vi "Cycle Complete.vi"(8 "error in (no error)":errorcluster, 11 "Active in":refnum<class "Active.lvclass">) -> (0 "error out":errorcluster, 3 "_State Machine Actor out":refnum<class "_State Machine Actor.lvclass">)   [LabVIEW 2024, in "Active.lvlib" / "Active.lvclass"]
uses:
  Active.lvclass
  Active.lvclass/Active.ctl
  Idle/Idle/Idle.lvclass
  C:/Users/uspoaotto/OneDrive - Oregon Tool/Desktop/working copies/stateMachineActor/src/Automation Controller/Automation Controller/Automation Controller.lvclass
  C:/Users/uspoaotto/OneDrive - Oregon Tool/Desktop/working copies/stateMachineActor/src/State Machine Actor/State Machine Actor/State Machine Actor.lvclass
  C:/Users/uspoaotto/OneDrive - Oregon Tool/Desktop/working copies/stateMachineActor/src/_State Machine Actor/_State Machine Actor/_State Machine Actor.lvclass
  C:/Program Files (x86)/National Instruments/LabVIEW 2024/vi.lib/ActorFramework/Actor/Actor.lvclass
  C:/Users/uspoaotto/OneDrive - Oregon Tool/Desktop/working copies/stateMachineActor/src/Idle/Idle/Idle.lvclass
  _State Machine Actor/_State Machine Actor/_State Machine Actor.lvclass
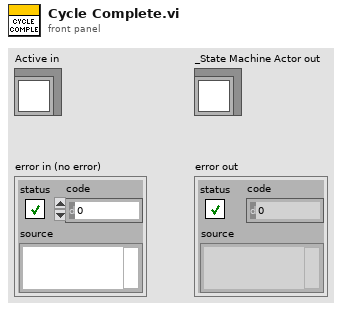
[diagram p1: front panel]
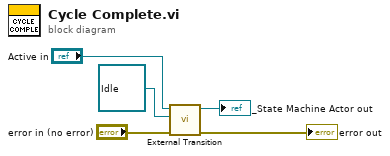
[diagram p0: block diagram]
diagram:
  n1 = call-dynamic "External Transition.vi"("error in (no error)"="error in (no error)", "Target State"=refnum<class "Idle.lvclass"> refnum ("Idle.lvlib:Idle.lvclass"), "State Machine Actor in"="Active in") -> ("error out"=→"error out":errorcluster, "_State Machine Actor out"=→"_State Machine Actor out":refnum<class "_State Machine Actor.lvclass">)  [unwired: 7 in]
